vi "Get Detector.vi"(10 "ypixels":i32, 11 "xpixels":i32) -> (1 "function return":u32, 2 "ypixels out":i32, 3 "xpixels out":i32)   [LabVIEW 2018, in "AndorSDK.lvlib"]
doc: "EXPNETTYPE unsigned int WINAPI GetDetector(int * xpixels, int * ypixels);"
uses:
  AndorSDK.lvlib
  ATMCD32D.dll
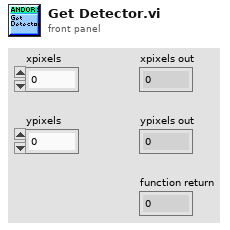
[diagram p1: front panel]
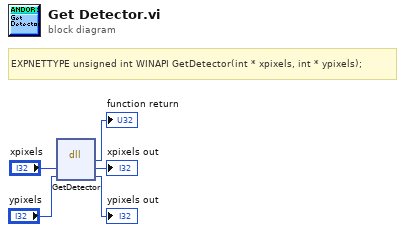
[diagram p0: block diagram]
diagram:
  # "EXPNETTYPE unsigned int WINAPI GetDetector(int * xpixels, int * ypixels);"
  n1 = dll-call lib="PTH2babs E\nPersönliches02 - Arbeit03-HiwijobsLabviewCodelibANDOR\tAndor SDK\nATMCD32D.*" fn="GetDetector"("xpixels"="xpixels", "ypixels"="ypixels") -> (→"function return":u32, "xpixels"=→"xpixels out":i32, "ypixels"=→"ypixels out":i32)  [unwired: 3 in, 2 out]
